vi "getName.vi"(8 "error in (no error)":errorcluster, 11 "car in":refnum<class "car.lvclass">) -> (0 "error out":errorcluster, 2 "name":string, 3 "car out":refnum<class "car.lvclass">)   [LabVIEW 2011, in "car.lvclass"]
uses:
  car.lvclass
  vehicleGeneric.lvclass
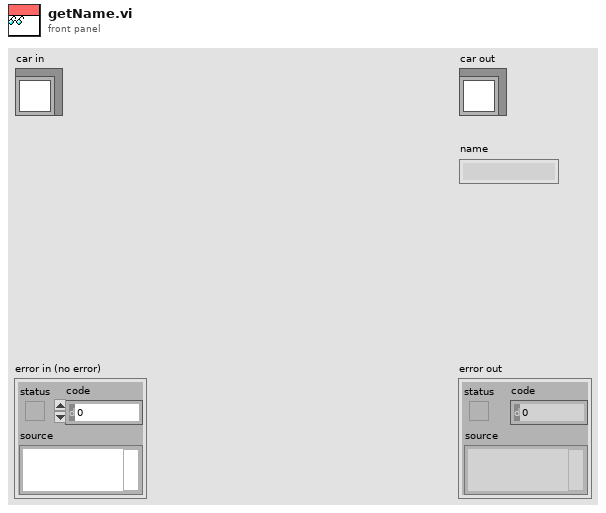
[diagram p1: front panel]
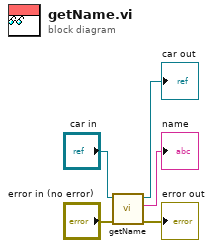
[diagram p0: block diagram]
diagram:
  n1 = call-parent "getName.vi"("error in (no error)"="error in (no error)", "vehicleGeneric in"="car in") -> ("error out"=→"error out":errorcluster, "name"=→"name":string, "vehicleGeneric out"=→"car out":refnum<class "car.lvclass">)  [unwired: 7 in]
